vi "Periodic Tasks.vi"(8 "error in":errorcluster) -> ()   [LabVIEW 2014]
doc: "This VI runs in parallel to other tasks. It can contain as many user-defined periodic loops as you need. These can carry out PID or other sorts of timed response."
uses:
  <vilib>/Rock Robotics/WPI/Joystick/WPI_JoystickGetSetRefNum.vi
  <vilib>/Rock Robotics/WPI/RobotDrive/WPI_RobotDriveGetSetRefNum.vi
  Robot Global Data.vi
  <vilib>/addons/control/pid/pid.llb/PID (DBL).vi
  <vilib>/addons/control/pid/NI_PID_pid.lvlib
panel:
  in  "CLAW_Neutral_Position":dbl=2.5 format="%#_13g"
  in  "Max_Analog_Volts":dbl=5.0 format="%#_13g"
  in  "Arm_Extend_Limit":dbl(slide)=0.95 scale=1.0..-1.0
  in  "Arm_Retract_Limit":dbl(slide)=-0.85 scale=1.0..-1.0
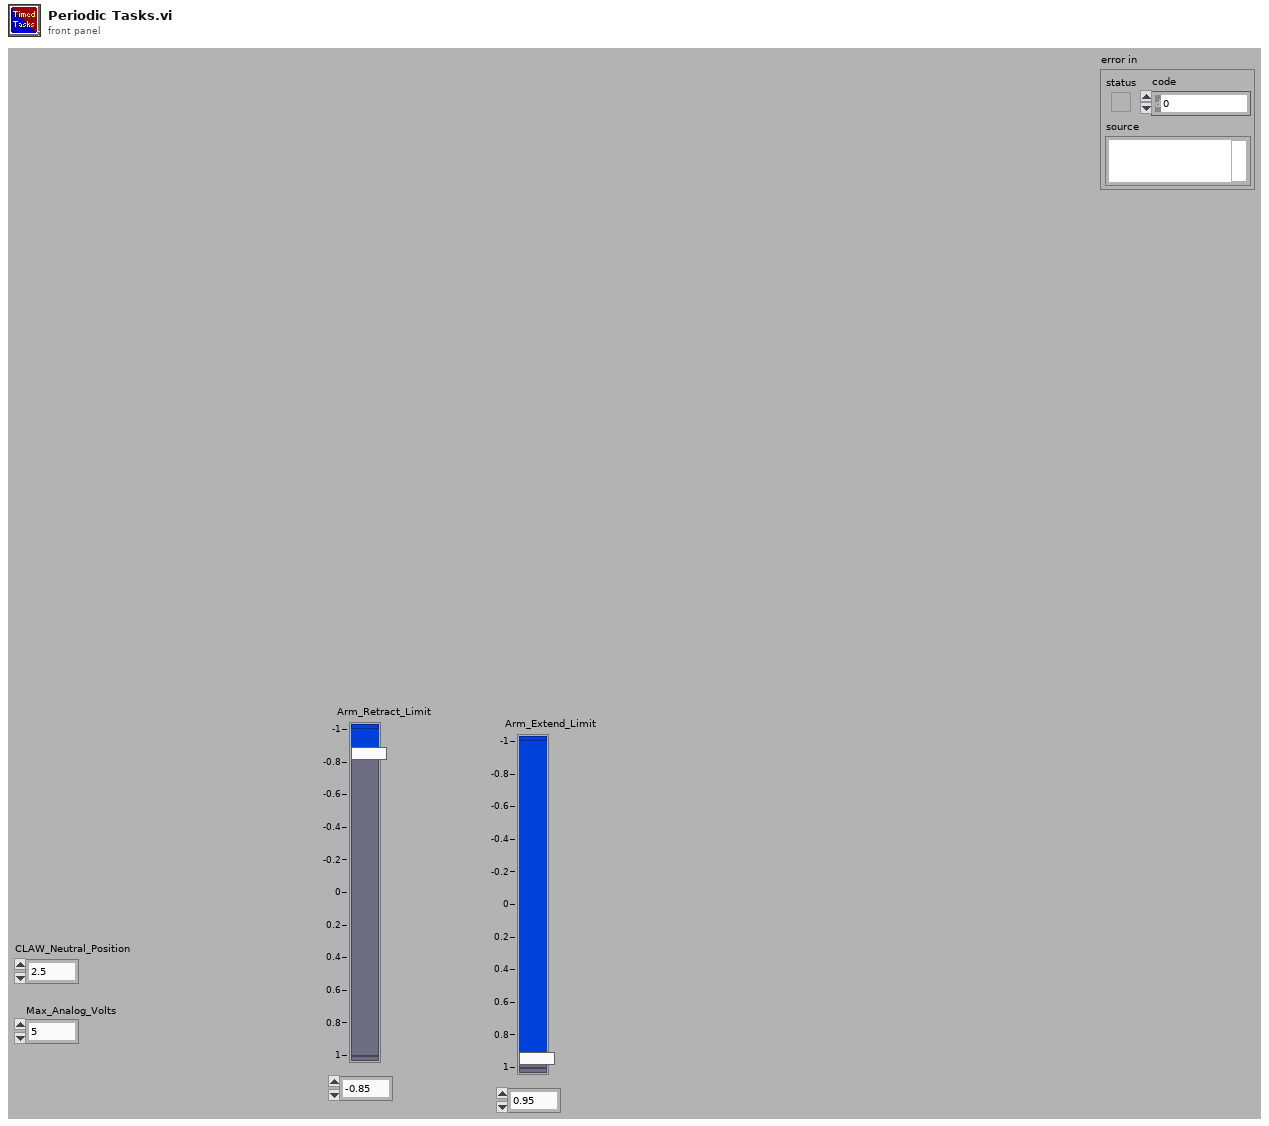
[diagram p1: front panel]
types:
  T1 = typedef "WPI_AnalogChannelDevRef.ctl" = cluster{"DevStatus":errorcluster, "Controller":T2, "Analog Channel":T3}
  T2 = typedef "FPGA_TypedefAnalogModule.ctl" = enum16{"Controller 1"}
  T3 = typedef "FPGA_AIChannel.ctl" = enum8{"AI 0", "AI 1", "AI 2", "AI 3", "AI MXP 0", "AI MXP 1", "AI MXP 2", "AI MXP 3", "Invalid"}
  T4 = typedef "WPI_MotorControlDeviceRef.ctl" = cluster{"DeviceStatus":errorcluster, "Type":T5, "PWM":cluster{"Controller":T6, "PWM Channel":T7, "DeadBand":T8}, "CAN":cluster{"Device Number":u8, "Control Mode":T9, "Semaphore":T10, "Max Vout":dbl, "TalonSRX Control Mode":T11}, "Invert":bool, "TransformRef":T12, "InvTransformRef":T12}
  T5 = typedef "WPI_MotorControlType.ctl" = enum16{"PWM", "CAN", "CANTalonSRX"}
  T6 = typedef "FPGA_TypedefDigitalModule.ctl" = enum16{"Controller 1"}
  T7 = typedef "FPGA_DIOPWMChannel.ctl" = enum8{"PWM 0", "PWM 1", "PWM 2", "PWM 3", "PWM 4", "PWM 5", "PWM 6", "PWM 7", "PWM 8", "PWM 9", "PWM MXP 0", "PWM MXP 1", "PWM MXP 2", "PWM MXP 3", "PWM MXP 4", "PWM MXP 5", "PWM MXP 6", "PWM MXP 7", "PWM MXP 8", "PWM MXP 9", "Invalid"}
  T8 = typedef "WPI_PWMDeadband.ctl" = cluster{"Name":string, "maxPositivePwm":i32, "minPositivePwm":i32, "centerPwm":i32, "maxNegativePwm":i32, "minNegativePwm":i32, "angularRange":u16}
  T9 = typedef "WPI_CANJaguar_ControlMode.ctl" = enum8{"Percent VBus", "Current", "Speed", "Position", "Voltage"}
  T10 = typedef "Semaphore RefNum" = refnum<k1>
  T11 = typedef "WPI_CANTalonSRX_APIControlMode.ctl" = enum8{"Percent VBus", "Speed", "Position", "Slave", "Unchanged / Invalid"}
  T12 = typedef "WPI_PWMTransform_ConPane.ctl" = refnum<vi>
  T13 = typedef "WPI_JoystickDevRef.ctl" = cluster{"Device":T14}
  T14 = typedef "WPI_JoystickDeviceEnum.ctl" = enum16{"USB 0", "USB 1", "USB 2", "USB 3", "USB 4", "USB 5"}
  T15 = typedef "WPI_RobotDriveDevRef.ctl" = cluster{"DevStatus":errorcluster, "Motors[]":T4[], "Square Inputs":bool, "Max Output":dbl}
  T16 = cluster{"JoystickDevRef":T13, "RobotDriveDevRef":T15}
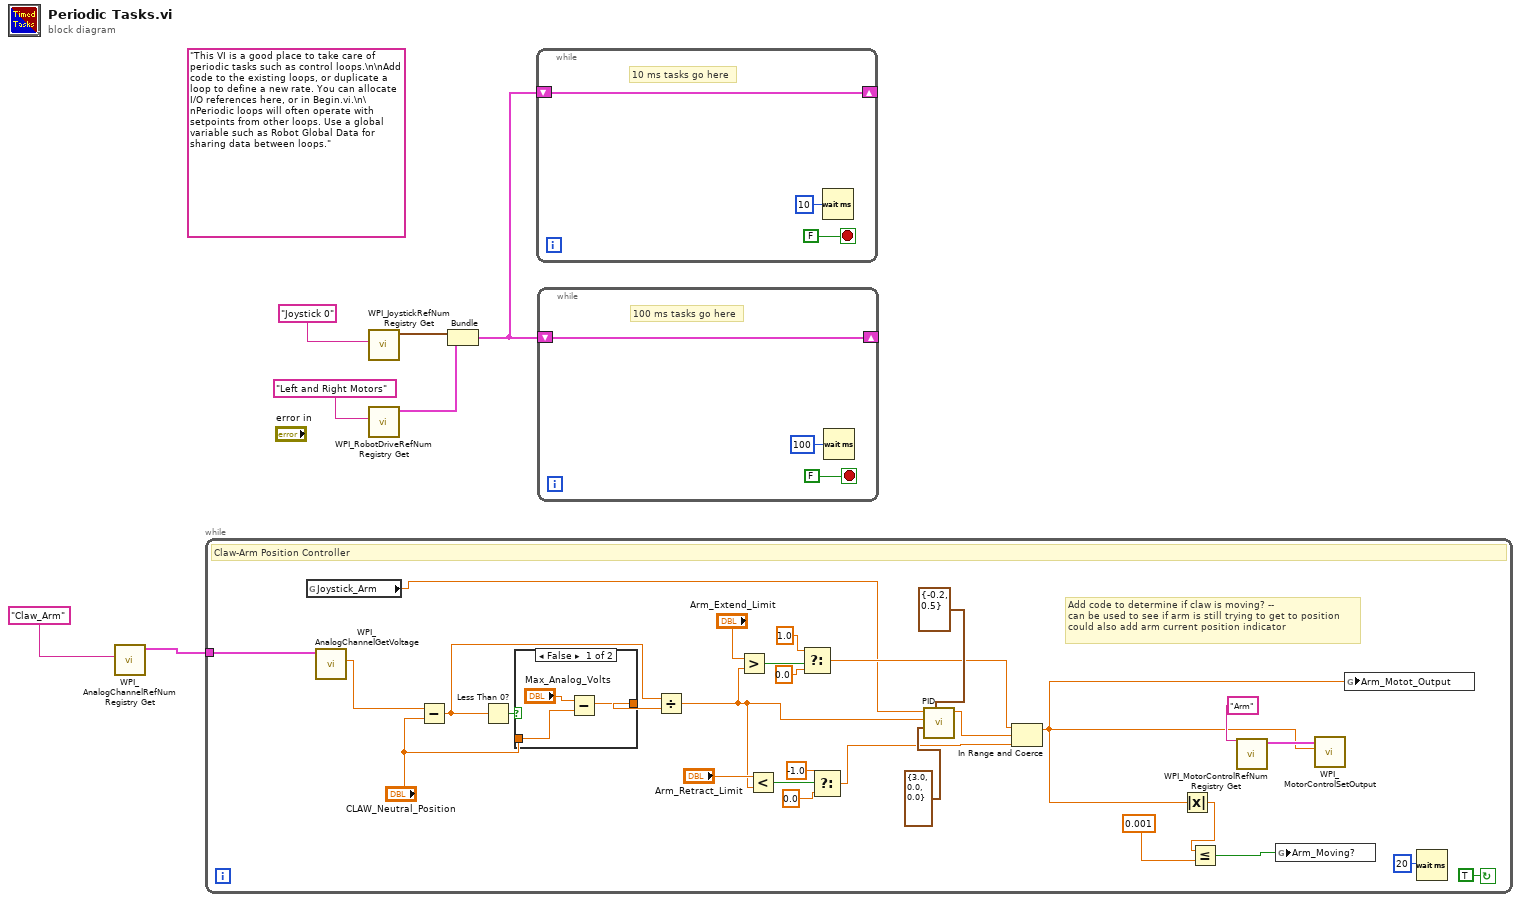
[diagram p0: block diagram]
diagram:
  (unwired) "This VI is a good place to take care of periodic tasks such as control loops.\n\nAdd code to the existing loops, or duplicate a loop to define a new rate. You can allocate I/O references here, or in Begin.vi.\n\nPeriodic loops will often operate with setpoints from other loops. Use a global variable such as Robot Global Data for sharing data between loops."
  n1 = call <vilib>:"WPI_AnalogChannelRefNum Registry Get.vi"("refnum name"="Claw_Arm") -> ("AIDeviceRef"=w1:T1)  [unwired: 1 in, 9 out]
  n2 = while {
    tunnel: w1 -> [w36]
    stop <- TRUE continue-if-true
    # "Add code to determine if claw is moving? -- \ncan be used to see if arm is still trying to get to position\ncould also add arm current position indicator"
    # "Claw-Arm Position Controller"
    n3 = global read "Robot Global Data.vi" "Joystick_Arm"() -> (w10:dbl)
    n4 = call <vilib>:"WPI_AnalogChannelGetVoltage.vi"("AIDeviceRef"=w36) -> ("Voltage"=w35:dbl)  [unwired: 1 in, 9 out]
    n5 = Subtract(x=w35, y="CLAW_Neutral_Position") -> (x-y=w27:dbl)
    n6 = Less Than 0?(x=w27) -> (x < 0?=w32:bool)
    n7 = case shown="False" w32 {
      tunnel: "CLAW_Neutral_Position" -> [w38 w40]
      tunnel: [w37 w40] -> w34
      frame False {
        n8 = Subtract(x="Max_Analog_Volts", y=w38) -> (x-y=w37:dbl)
      }
      frame True {
      }
    }
    n9 = Divide(x=w27, y=w34) -> (x/y=w18:dbl)
    n10 = Greater?(x="Arm_Extend_Limit", y=w18) -> (0:w25:bool)
    n11 = Less?(x="Arm_Retract_Limit", y=w18) -> (x < y?=w22:bool)
    n12 = Select(t=1.0, s=w25, f=0.0) -> (s? t:f=w16:dbl)
    n13 = Select(t=-1.0, s=w22, f=0.0) -> (s? t:f=w15:dbl)
    n14 = call-poly <vilib>:"PID.vi"("output range"=cluster{"output low":dbl, "output high":dbl} {"output low"=-0.2, "output high"=0.5}, "PID gains"=cluster{dbl, dbl, dbl} {3.0, 0.0, 0.0}, "process variable"=w18, "setpoint"=w10) -> ("output"=w17:dbl)  [unwired: 2 in, 5 out]
    n15 = In Range and Coerce(upper limit=w16, x=w17, lower limit=w15) -> (coerced(x)=w9:dbl)  [unwired: 1 out]
    n16 = Absolute Value(x=w9) -> (abs(x)=w11:dbl)
    n17 = Less Or Equal?(x=w11, y=0.001) -> (x <= y?=w8:bool)
    n18 = call <vilib>:"WPI_MotorControlRefNum Registry Get.vi"("refnum name"="Arm") -> ("MotorControlDevRef"=w30:T4)  [unwired: 1 in, 9 out]
    n19 = global write "Robot Global Data.vi" "Arm_Moving?"(w8) -> ()
    n20 = call <vilib>:"WPI_MotorControlSetOutput.vi"("Output"=w9, "MotorControlDevRef"=w30) -> ()  [unwired: 2 in, 8 out]
    n21 = global write "Robot Global Data.vi" "Arm_Motot_Output"(w9) -> ()
    n22 = Wait (ms)(milliseconds to wait=20) -> ()  [unwired: 1 out]
  }
  n23 = call <vilib>:"WPI_JoystickRefNum Registry Get.vi"("refnum name"="Joystick 0") -> ("JoystickDevRef"=w5:T13)  [unwired: 1 in, 9 out]
  n24 = call <vilib>:"WPI_RobotDriveRefNum Registry Get.vi"("refnum name"="Left and Right Motors") -> ("RobotDriveDevRef"=w4:T15)  [unwired: 1 in, 9 out]
  n25 = Bundle("JoystickDevRef"=w5, "RobotDriveDevRef"=w4) -> (w3:T16)  [unwired: 1 out]
  n26 = while {
    shift-right: [w41] -> _
    shift-left: w3 -> [w41]
    stop <- FALSE stop-if-true
    # "10 ms tasks go here"
    n27 = Wait (ms)(milliseconds to wait=u32 10) -> ()  [unwired: 1 out]
  }
  n28 = while {
    shift-right: [w44] -> _
    shift-left: w3 -> [w44]
    stop <- FALSE stop-if-true
    # "100 ms tasks go here"
    n29 = Wait (ms)(milliseconds to wait=u32 100) -> ()  [unwired: 1 out]
  }
